vi "Configure Modulation Low Level (PWM Frequency).vi"(8 "error in":errorcluster, 10 "Modulation Frequency (10 Hz)":dbl=10.0, 11 "VISA resource name":refnum<visa-resource-name>) -> (0 "error out":errorcluster, 3 "VISA resource name out":refnum<visa-resource-name>)   [LabVIEW 2017, in "Keithley 3390.lvlib"]
doc: "Sets the frequency of the internal modulating source signal."
uses:
  Keithley 3390.lvlib
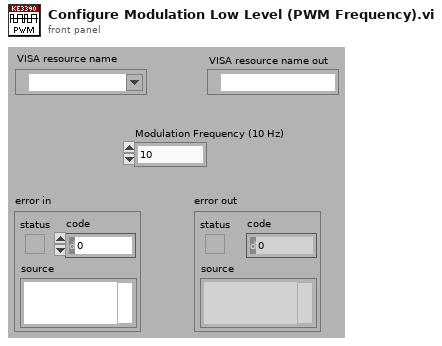
[diagram p1: front panel]
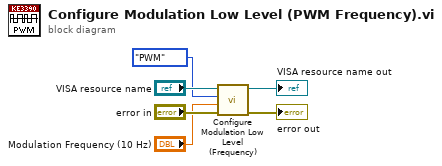
[diagram p0: block diagram]
diagram:
  n1 = call "Configure Modulation Low Level (Frequency).vi"("error in (no error)"="error in", "Frequency (100.00 Hz)"="Modulation Frequency (10 Hz)", "Modulation (AM)"=enum16{"AM", "FM", "PM", "FSK", "PWM"}."PWM" ("Modulation (0:AM)"), "VISA resource name"="VISA resource name") -> ("error out"=→"error out":errorcluster, "VISA resource name out"=→"VISA resource name out":refnum<visa-resource-name>)  [unwired: 6 in]
